vi "ReadAvs47b.vi"(6 "STABILISATION DELAY (ms)":i32, 7 "SYNCHRONISE TO ADC":bool=TRUE, 8 "LV ERROR IN":errorcluster, 11 "CONFIGURATION CLUSTER":T1) -> (0 "LV ERROR OUT":errorcluster, 1 "ADC":i32, 2 "RESISTANCE (OHMS)":sgl, 3 "MODIFIED CONFIGURATION CLUSTER":T1, 4 "WAITING FOR AL":bool, 5 "ADC OVERRANGE":bool)   [LabVIEW 2023]
doc: "Reads the last or next ADC result.\nReads the configuration of the bridge\n(useful in local mode)"
panel:
  # "ReadAvs47b.vi"
  # "This VI configures the AVS-47B (but not the TS-530A).  The stabilisation delay can be zero if  the bridge has been\nconfigured earlier using SendConfigurationToAvs47b.vi or if it has been configured by an earlier reading and\nno changes have been made since then.  Using the stabilisation delay with each reading makes the system very\nslow and is not necessary. \n\nThe VI reads from the bridge its current setup and the A/D converter's output.  A new setup is sent to the bridge\nregardless of the local/remote mode, but if the configuration clusters says \"local\", the bridge does not \nchange its state.\n\nIf \"synchronise to ADC\" is false, this VI reads the result that is available from the bridge.  The age of the result\nmay vary from 0 to 400 milliseconds but the reading is obtained immediately. Without synchronisation, \na fast application program can read the same result many times.\n\nIf \"synchronise to ADC\" is true, this VI transacts with the bridge, resetting its Alarm (AL) output. Then the \nprogram enters into a while-loop, polling the AL signal at 5 millisecond intervals.  The AVS-47B sets AL true\nas soon as the next A/D conversion has completed. When this happens, the program exits the while loop,\nwaits a little and reads the ADC result and bridge settings.\n\nIf AL is not encountered, the \"waiting for AL\" indicator is continuously on. This can be due to a cable fault\nor if a wrong port has been opened as the VISA resource. \n\nDuring ADC overrange (input to ADC > 2 Volts), the overrange indicator turns red and the ADC and resistance\nindicators show zero.   LabView may show error if no VISA session has been opened."
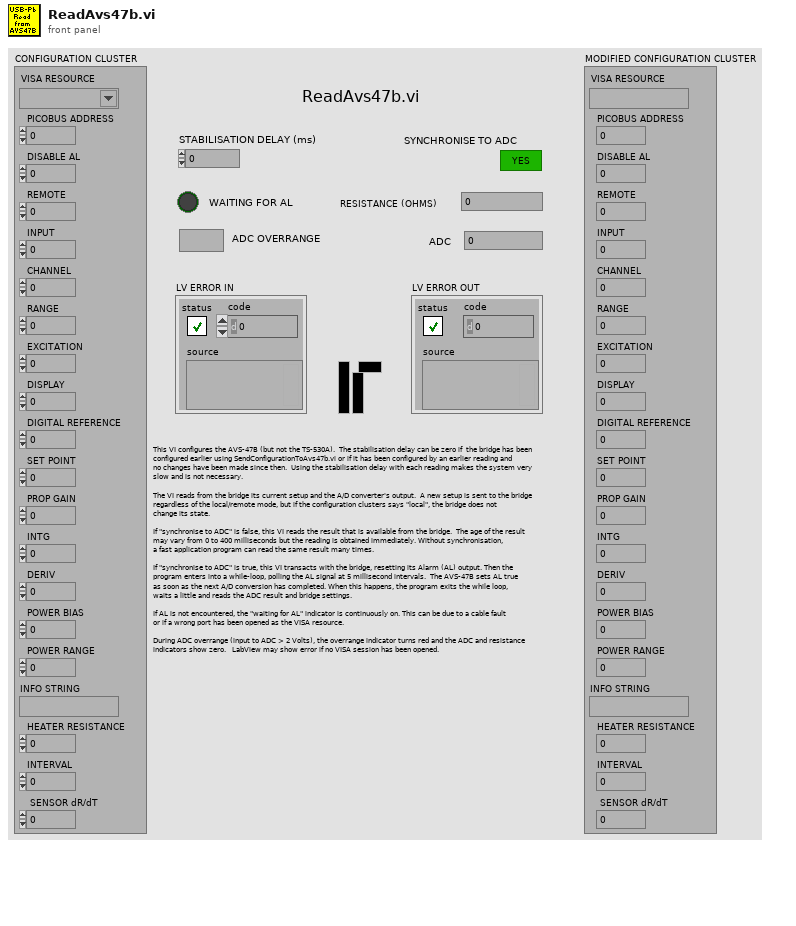
[diagram p1: front panel]
types:
  T1 = cluster{"VISA RESOURCE":refnum<visa-resource-name>, "PICOBUS ADDRESS":u8, "DISABLE AL":u8, "REMOTE":u8, "INPUT":u8, "CHANNEL":u8, "RANGE":u8, "EXCITATION":u8, "DISPLAY":u8, "DIGITAL REFERENCE":u16, "SET POINT":dbl, "PROP GAIN":u8, "INTG":u8, "DERIV":u8, "POWER BIAS":u8, "POWER RANGE":u8, "INFO STRING":string, "HEATER RESISTANCE":dbl, "INTERVAL":u8, " SENSOR dR/dT":u8}
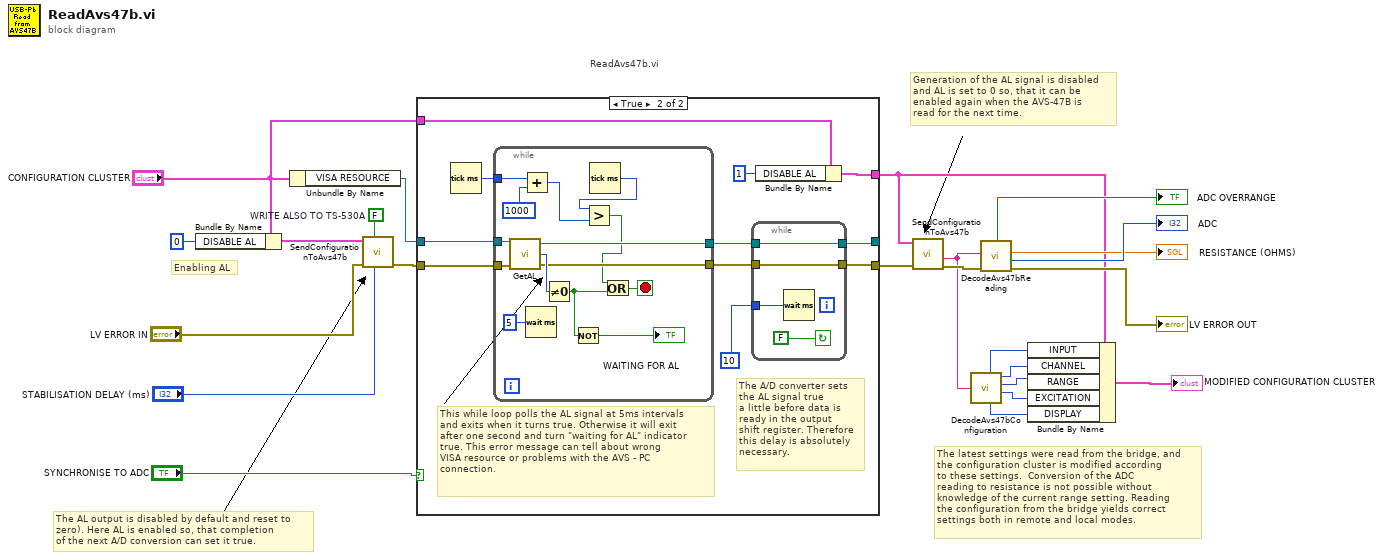
[diagram p0: block diagram]
diagram:
  w23 = FALSE  # WRITE ALSO TO TS-530A
  # "Generation of the AL signal is disabled\nand AL is set to 0 so, that it can be \nenabled again when the AVS-47B is\nread for the next time."
  # "The latest settings were read from the bridge, and\nthe configuration cluster is modified according\nto these settings.  Conversion of the ADC\nreading to resistance is not possible without\nknowledge of the current range setting. Reading\nthe configuration from the bridge yields correct\nsettings both in remote and local modes."
  # "The AL output is disabled by default and reset to\nzero). Here AL is enabled so, that completion \nof the next A/D conversion can set it true."
  # "ReadAvs47b.vi"
  # "Enabling AL"
  n1 = Bundle By Name(cluster="CONFIGURATION CLUSTER", "DISABLE AL"=u8 0) -> (w19:T1)
  n2 = Unbundle By Name("CONFIGURATION CLUSTER") -> ("VISA RESOURCE"=w21:refnum<visa-resource-name>)
  n3 = call "SendConfigurationToAvs47b.vi"("STABILISATION DELAY (ms)"="STABILISATION DELAY (ms)", "WRITE ALSO TO TS-530A"=w23, "LV ERROR IN"="LV ERROR IN", "CONFIGURATION CLUSTER"=w19) -> ("LV ERROR OUT"=w22:errorcluster)  [unwired: 4 in, 3 out]
  n4 = case shown="True" "SYNCHRONISE TO ADC" {
    tunnel: w21 -> [w26 w35]
    tunnel: w22 -> [w25 w34]
    tunnel: [w26 w31] -> _
    tunnel: [w25 w30] -> w8
    tunnel: "CONFIGURATION CLUSTER" -> [w24 w28]
    tunnel: [w24 w27] -> w7
    frame False {
      # "This case is run, if \"synchronise to ADC\" is false.\nThe reading is taken immediately regardless of its\nage or whether it has already been read earlier."
    }
    frame True {
      # "This while loop polls the AL signal at 5ms intervals\nand exits when it turns true. Otherwise it will exit\nafter one second and turn \"waiting for AL\" indicator\ntrue. This error message can tell about wrong\nVISA resource or problems with the AVS - PC \nconnection."
      # "The A/D converter sets\nthe AL signal true\na little before data is\nready in the output\nshift register. Therefore\nthis delay is absolutely\nnecessary."
      n5 = Tick Count (ms)() -> (millisecond timer value=w37:u32)
      n6 = while {
        tunnel: w34 -> [w53]
        tunnel: w35 -> [w52]
        tunnel: [w51] -> w32
        tunnel: [w50] -> w33
        tunnel: w37 -> [w49]
        stop <- w45 stop-if-true
        n7 = call "GetAL.vi"("error in (no error)"=w53, "VISA resource"=w52) -> ("error out"=w51:errorcluster, "AL(=DSR) State"=w55:i16, "dup VISA resource"=w50:refnum<visa-resource-name>)  [unwired: 1 in]
        n8 = Add(x=w49, y=u32 1000) -> (x+y=w46:u32)
        n9 = Wait (ms)(milliseconds to wait=5) -> ()  [unwired: 1 out]
        n10 = Not Equal To 0?(x=w55) -> (x != 0?=w43:bool)
        n11 = Not(x=w43) -> (.not. x?=→"WAITING FOR AL":bool)
        n12 = Tick Count (ms)() -> (millisecond timer value=w47:u32)
        n13 = Greater?(x=w47, y=w46) -> (0:w44:bool)
        n14 = Or(x=w44, y=w43) -> (x .or. y?=w45:bool)
      }
      n15 = while {
        tunnel: 10 -> [w40]
        tunnel: w33 -> [w39]
        tunnel: w32 -> [w38]
        tunnel: [w39] -> w31
        tunnel: [w38] -> w30
        stop <- FALSE continue-if-true
        n16 = Wait (ms)(milliseconds to wait=w40) -> ()  [unwired: 1 out]
      }
      n17 = Bundle By Name(cluster=w28, "DISABLE AL"=u8 1) -> (w27:T1)
    }
  }
  n18 = call "SendConfigurationToAvs47b.vi"("LV ERROR IN"=w8, "CONFIGURATION CLUSTER"=w7) -> ("LV ERROR OUT"=w6:errorcluster, "AVS47B RXSTR"=w4:string)  [unwired: 6 in, 2 out]
  n19 = call "DecodeAvs47bConfiguration.vi"("RXSTR"=w4) -> ("INPUT OUT"=w14:u16, "CHANNEL OUT"=w13:u16, "RANGE OUT"=w12:u16, "DISPLAY OUT"=w10:u16, "EXCITATION OUT"=w11:u16)  [unwired: 5 in]
  n20 = call "DecodeAvs47bReading.vi"("LV ERROR IN"=w6, "RXSTR"=w4) -> ("LV ERROR OUT"=→"LV ERROR OUT":errorcluster, "ADC"=→"ADC":i32, "RESISTANCE"=→"RESISTANCE (OHMS)":sgl, "ADC OVERRANGE"=→"ADC OVERRANGE":bool)  [unwired: 4 in, 2 out]
  n21 = Bundle By Name(cluster=w7, "INPUT"=w14, "CHANNEL"=w13, "RANGE"=w12, "EXCITATION"=w11, "DISPLAY"=w10) -> (→"MODIFIED CONFIGURATION CLUSTER":T1)
